vi "test-Implicit-Model-Follower-Test2.vi"(8 "error in (no error)":errorcluster) -> (0 "error out":errorcluster, 3 "All tests passed":bool)   [LabVIEW 2019]
uses:
  <vilib>/Rock Robotics/WPI/ThirdParty/JAS_Junk/TrajLib/LinearSystem_New.vi
  <vilib>/Rock Robotics/WPI/ThirdParty/JAS_Junk/TrajLib/MatBuilder_Create.vi
  <vilib>/Rock Robotics/WPI/ThirdParty/JAS_Junk/TrajLib/MatrixHelper_Zero.vi
  <vilib>/Rock Robotics/WPI/ThirdParty/JAS_Junk/TrajLib/Discretization_DiscretizeAB.vi
  <vilib>/Analysis/baseanly.llb/A x B.vi
  <vilib>/Analysis/baseanly.llb/Real A x B.vi
  <vilib>/Rock Robotics/WPI/ThirdParty/JAS_Junk/TrajLib/MatrixHelper_CoerceSize.vi
  <vilib>/Rock Robotics/WPI/ThirdParty/JAS_Junk/TrajLib/Matrix_Exp.vi
  <vilib>/Rock Robotics/WPI/ThirdParty/JAS_Junk/TrajLib/Matrix_AssignBlock.vi
  <vilib>/Rock Robotics/WPI/ThirdParty/JAS_Junk/TrajLib/Matrix_ExtractFrom.vi
  <vilib>/Analysis/7linalg.llb/Matrix Exp.vi
  <vilib>/Analysis/7linalg.llb/Real Matrix Exp.vi
  <vilib>/Analysis/Matrix/Numeric/Multiply/Multiply.vi
  <vilib>/Analysis/Matrix/Numeric/Multiply/Multiply - RM,R.vi
  <vilib>/Analysis/Matrix/Numeric/Add/Add.vi
  <vilib>/Analysis/Matrix/Numeric/Add/Add - RM,RM.vi
  <vilib>/Rock Robotics/WPI/ThirdParty/JAS_Junk/TrajLib/Trajectory_Library.lvlib
panel:
  out "Test 3":bool
  out "Test 2":bool
  out "Test 1":bool
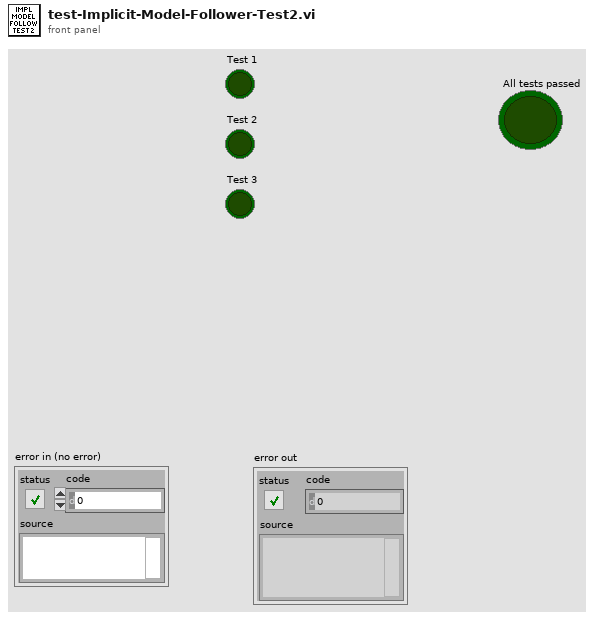
[diagram p1: front panel]
types:
  T1 = typedef "NI_Matrix.lvlib/RealMatrix.ctl" = dbl[][]
  T2 = typedef "Trajectory_Library.lvlib/LINEAR_SYSTEM.ctl" = cluster{"m_A":T1, "m_B":T1, "m_C":T1, "m_D":T1, "States":i32, "Inputs":i32, "Outputs":i32}
  T3 = typedef "Trajectory_Library.lvlib/IMPLICIT_MODEL_FOLLOWER.ctl" = cluster{"m_A":T1, "m_B":T1, "m_U":T1, "States":i32, "Inputs":i32}
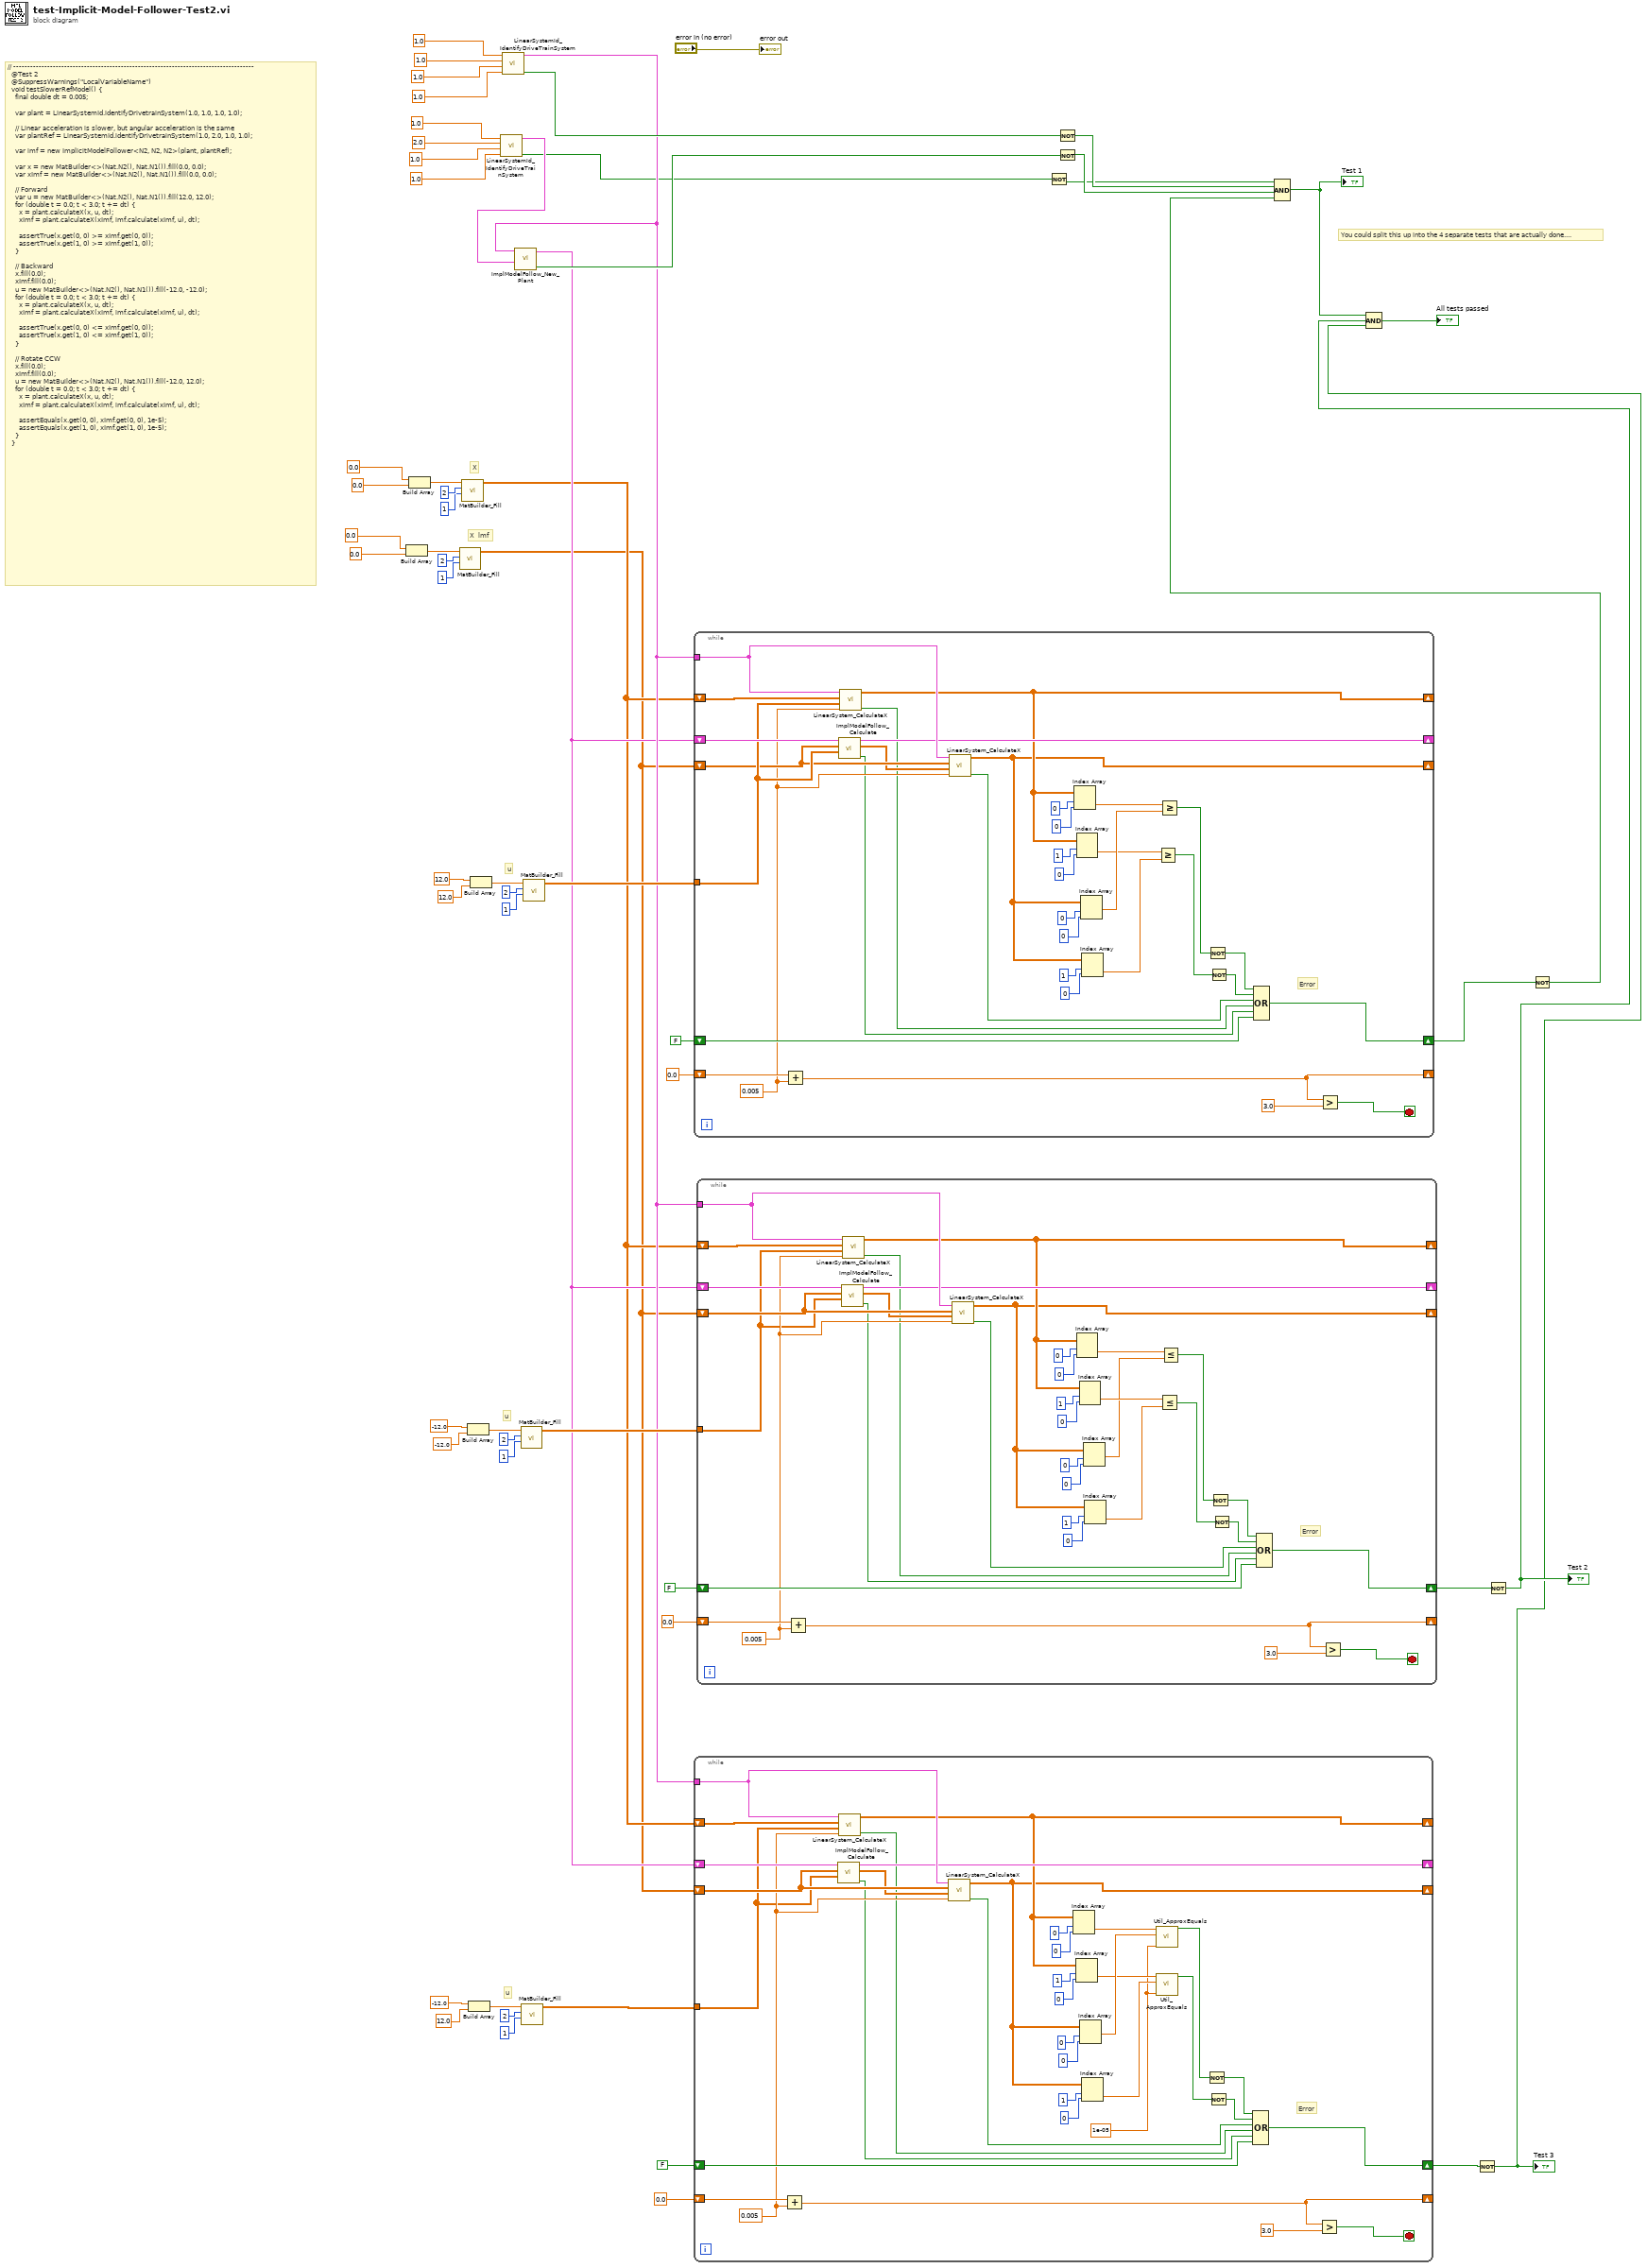
[diagram p0: block diagram]
diagram:
  # "// -------------------------------------------------------------------------------------\n  @Test 2\n  @SuppressWarnings(\"LocalVariableName\")\n  void testSlowerRefModel() {\n    final double dt = 0.005;\n\n    var plant = LinearSystemId.identifyDrivetrainSystem(1.0, 1.0, 1.0, 1.0);\n\n    // Linear acceleration is slower, but angular acceleration is the same\n    var plantRef = LinearSystemId.identifyDrivetrainSystem(1.0, 2.0, 1.0, 1.0);\n\n    var imf = new ImplicitModelFollower<N2, N2, N2>(plant, plantRef);\n\n    var x = new MatBuilder<>(Nat.N2(), Nat.N1()).fill(0.0, 0.0);\n    var xImf = new MatBuilder<>(Nat.N2(), Nat.N1()).fill(0.0, 0.0);\n\n    // Forward\n    var u = new MatBuilder<>(Nat.N2(), Nat.N1()).fill(12.0, 12.0);\n    for (double t = 0.0; t < 3.0; t += dt) {\n      x = plant.calculateX(x, u, dt);\n      xImf = plant.calculateX(xImf, imf.calculate(xImf, u), dt);\n\n      assertTrue(x.get(0, 0) >= xImf.get(0, 0));\n      assertTrue(x.get(1, 0) >= xImf.get(1, 0));\n    }\n\n    // Backward\n    x.fill(0.0);\n    xImf.fill(0.0);\n    u = new MatBuilder<>(Nat.N2(), Nat.N1()).fill(-12.0, -12.0);\n    for (double t = 0.0; t < 3.0; t += dt) {\n      x = plant.calculateX(x, u, dt);\n      xImf = plant.calculateX(xImf, imf.calculate(xImf, u), dt);\n\n      assertTrue(x.get(0, 0) <= xImf.get(0, 0));\n      assertTrue(x.get(1, 0) <= xImf.get(1, 0));\n    }\n\n    // Rotate CCW\n    x.fill(0.0);\n    xImf.fill(0.0);\n    u = new MatBuilder<>(Nat.N2(), Nat.N1()).fill(-12.0, 12.0);\n    for (double t = 0.0; t < 3.0; t += dt) {\n      x = plant.calculateX(x, u, dt);\n      xImf = plant.calculateX(xImf, imf.calculate(xImf, u), dt);\n\n      assertEquals(x.get(0, 0), xImf.get(0, 0), 1e-5);\n      assertEquals(x.get(1, 0), xImf.get(1, 0), 1e-5);\n    }\n  }"
  # "X  lmf"
  # "You could split this up into the 4 separate tests that are actually done...."
  # "u"
  # "u"
  # "u"
  # "X"
  n1 = Build Array(0.0 ("element"), 0.0 ("element")) -> (w31:dbl[])
  n2 = Build Array(0.0 ("element"), 0.0 ("element")) -> (w57:dbl[])
  n3 = call <vilib>:"MatBuilder_Fill.vi"("Columns"=1, "Rows"=2, "Value List"=w31) -> ("output matrix"=w11:T1)  [unwired: 8 in]
  n4 = call <vilib>:"MatBuilder_Fill.vi"("Columns"=1, "Rows"=2, "Value List"=w57) -> ("output matrix"=w12:T1)  [unwired: 8 in]
  n5 = Build Array(-12.0 ("element"), -12.0 ("element")) -> (w41:dbl[])
  n6 = Build Array(-12.0 ("element"), 12.0 ("element")) -> (w36:dbl[])
  n7 = Build Array(12.0 ("element"), 12.0 ("element")) -> (w51:dbl[])
  n8 = call <vilib>:"LinearSystemId_IdentifyDriveTrainSystem.vi"("kAAngular"=1.0 ("rbMeters"), "kVAngular"=1.0 ("rMeters"), "kALinear"=2.0 ("MassKg"), "kVLinear"=1.0 ("JKgMetersSquared")) -> ("Size Coerced"=w1:bool, "Linearsystem"=w3:T2)  [unwired: 6 in]
  n9 = call <vilib>:"LinearSystemId_IdentifyDriveTrainSystem.vi"("kAAngular"=1.0 ("rbMeters"), "kVAngular"=1.0 ("rMeters"), "kALinear"=1.0 ("MassKg"), "kVLinear"=1.0 ("JKgMetersSquared")) -> ("Size Coerced"=w52:bool, "Linearsystem"=w14:T2)  [unwired: 6 in]
  n10 = call <vilib>:"ImplModelFollow_New_Plant.vi"("PlantRef"=w3, "Plant"=w14) -> ("Error"=w26:bool, "IMPLICIT_MODEL_FOLLOWER"=w13:T3)  [unwired: 8 in]
  n11 = call <vilib>:"MatBuilder_Fill.vi"("Columns"=1, "Rows"=2, "Value List"=w41) -> ("output matrix"=w19:T1)  [unwired: 8 in]
  n12 = call <vilib>:"MatBuilder_Fill.vi"("Columns"=1, "Rows"=2, "Value List"=w36) -> ("output matrix"=w15:T1)  [unwired: 8 in]
  n13 = call <vilib>:"MatBuilder_Fill.vi"("Columns"=1, "Rows"=2, "Value List"=w51) -> ("output matrix"=w45:T1)  [unwired: 8 in]
  n14 = while {
    shift-right: [w95] -> _
    shift-left: 0.0 -> [w98]
    tunnel: w14 -> [w85]
    shift-right: [w74] -> _
    shift-left: w12 -> [w94]
    shift-right: [w82] -> w8
    shift-left: FALSE -> [w83]
    shift-right: [w73] -> _
    shift-left: w11 -> [w79]
    shift-right: [w80] -> _
    shift-left: w13 -> [w81]
    tunnel: w15 -> [w64]
    stop <- w97 stop-if-true
    w63 = 1e-05 ("Tolerance")
    w77 = 0.005
    # "Error"
    n15 = Add(x=w98, y=w77) -> (x+y=w95:dbl)
    n16 = call <vilib>:"ImplModelFollow_Calculate.vi"("U"=w64, "X"=w79, "in IMPLICIT_MODEL_FOLLOWER"=w81) -> ("Error"=w75:bool, "U Out"=w78:T1, "out IMPLICIT_MODEL_FOLLOWER"=w80:T3)  [unwired: 6 in]
    n17 = call <vilib>:"LinearSystem_CalculateX.vi"("dT_Seconds"=w77, "ClampedU"=w64, "X"=w94, "Linearsystem"=w85) -> ("Error"=w76:bool, "outX"=w74:T1)  [unwired: 6 in]
    n18 = call <vilib>:"LinearSystem_CalculateX.vi"("dT_Seconds"=w77, "ClampedU"=w78, "X"=w79, "Linearsystem"=w85) -> ("Error"=w84:bool, "outX"=w73:T1)  [unwired: 6 in]
    n19 = Index Array(array=w74, index (row)=0, index (col)=0) -> (element=w72:dbl)
    n20 = Index Array(array=w74, index (row)=1, index (col)=0) -> (element=w70:dbl)
    n21 = Index Array(array=w73, index (row)=0, index (col)=0) -> (element=w71:dbl)
    n22 = Index Array(array=w73, index (row)=1, index (col)=0) -> (element=w69:dbl)
    n23 = call <vilib>:"Util_ApproxEquals.vi"("Tolerance"=w63, "Value 2"=w71, "Value 1"=w72) -> ("ApproxEquals"=w66:bool)  [unwired: 8 in]
    n24 = call <vilib>:"Util_ApproxEquals.vi"("Tolerance"=w63, "Value 2"=w69, "Value 1"=w70) -> ("ApproxEquals"=w65:bool)  [unwired: 8 in]
    n25 = Not(x=w66) -> (.not. x?=w67:bool)
    n26 = Not(x=w65) -> (.not. x?=w68:bool)
    n27 = Compound Arithmetic op=OR(w67, w68, w84, w76, w75, w83) -> (w82:bool)
    n28 = Greater?(x=w95, y=3.0) -> (0:w97:bool)
  }
  n29 = while {
    shift-right: [w130] -> _
    shift-left: 0.0 -> [w133]
    tunnel: w14 -> [w120]
    tunnel: w45 -> [w115]
    shift-right: [w108] -> _
    shift-left: w12 -> [w129]
    shift-right: [w117] -> w43
    shift-left: FALSE -> [w118]
    shift-right: [w107] -> _
    shift-left: w11 -> [w113]
    shift-right: [w114] -> _
    shift-left: w13 -> [w116]
    stop <- w132 stop-if-true
    w111 = 0.005
    # "Error"
    n30 = Add(x=w133, y=w111) -> (x+y=w130:dbl)
    n31 = call <vilib>:"ImplModelFollow_Calculate.vi"("U"=w115, "X"=w113, "in IMPLICIT_MODEL_FOLLOWER"=w116) -> ("Error"=w109:bool, "U Out"=w112:T1, "out IMPLICIT_MODEL_FOLLOWER"=w114:T3)  [unwired: 6 in]
    n32 = call <vilib>:"LinearSystem_CalculateX.vi"("dT_Seconds"=w111, "ClampedU"=w115, "X"=w129, "Linearsystem"=w120) -> ("Error"=w110:bool, "outX"=w108:T1)  [unwired: 6 in]
    n33 = call <vilib>:"LinearSystem_CalculateX.vi"("dT_Seconds"=w111, "ClampedU"=w112, "X"=w113, "Linearsystem"=w120) -> ("Error"=w119:bool, "outX"=w107:T1)  [unwired: 6 in]
    n34 = Index Array(array=w108, index (row)=0, index (col)=0) -> (element=w104:dbl)
    n35 = Index Array(array=w108, index (row)=1, index (col)=0) -> (element=w101:dbl)
    n36 = Index Array(array=w107, index (row)=0, index (col)=0) -> (element=w103:dbl)
    n37 = Index Array(array=w107, index (row)=1, index (col)=0) -> (element=w100:dbl)
    n38 = Greater Or Equal?(x=w101, y=w100) -> (x >= y?=w99:bool)
    n39 = Greater Or Equal?(x=w104, y=w103) -> (x >= y?=w102:bool)
    n40 = Not(x=w102) -> (.not. x?=w105:bool)
    n41 = Not(x=w99) -> (.not. x?=w106:bool)
    n42 = Compound Arithmetic op=OR(w105, w106, w119, w110, w109, w118) -> (w117:bool)
    n43 = Greater?(x=w130, y=3.0) -> (0:w132:bool)
  }
  n44 = while {
    shift-right: [w165] -> _
    shift-left: 0.0 -> [w168]
    tunnel: w14 -> [w155]
    shift-right: [w144] -> _
    shift-left: w12 -> [w164]
    shift-right: [w152] -> w16
    shift-left: FALSE -> [w153]
    shift-right: [w143] -> _
    shift-left: w11 -> [w149]
    shift-right: [w150] -> _
    shift-left: w13 -> [w151]
    tunnel: w19 -> [w140]
    stop <- w167 stop-if-true
    w147 = 0.005
    # "Error"
    n45 = Add(x=w168, y=w147) -> (x+y=w165:dbl)
    n46 = call <vilib>:"ImplModelFollow_Calculate.vi"("U"=w140, "X"=w149, "in IMPLICIT_MODEL_FOLLOWER"=w151) -> ("Error"=w145:bool, "U Out"=w148:T1, "out IMPLICIT_MODEL_FOLLOWER"=w150:T3)  [unwired: 6 in]
    n47 = call <vilib>:"LinearSystem_CalculateX.vi"("dT_Seconds"=w147, "ClampedU"=w140, "X"=w164, "Linearsystem"=w155) -> ("Error"=w146:bool, "outX"=w144:T1)  [unwired: 6 in]
    n48 = call <vilib>:"LinearSystem_CalculateX.vi"("dT_Seconds"=w147, "ClampedU"=w148, "X"=w149, "Linearsystem"=w155) -> ("Error"=w154:bool, "outX"=w143:T1)  [unwired: 6 in]
    n49 = Index Array(array=w144, index (row)=0, index (col)=0) -> (element=w135:dbl)
    n50 = Index Array(array=w144, index (row)=1, index (col)=0) -> (element=w139:dbl)
    n51 = Index Array(array=w143, index (row)=0, index (col)=0) -> (element=w136:dbl)
    n52 = Index Array(array=w143, index (row)=1, index (col)=0) -> (element=w138:dbl)
    n53 = Less Or Equal?(x=w139, y=w138) -> (x <= y?=w137:bool)
    n54 = Less Or Equal?(x=w135, y=w136) -> (x <= y?=w134:bool)
    n55 = Not(x=w134) -> (.not. x?=w141:bool)
    n56 = Not(x=w137) -> (.not. x?=w142:bool)
    n57 = Compound Arithmetic op=OR(w141, w142, w154, w146, w145, w153) -> (w152:bool)
    n58 = Greater?(x=w165, y=3.0) -> (0:w167:bool)
  }
  n59 = Not(x=w1) -> (.not. x?=w2:bool)
  n60 = Not(x=w52) -> (.not. x?=w24:bool)
  n61 = Not(x=w26) -> (.not. x?=w25:bool)
  n62 = Not(x=w8) -> (.not. x?=w20:bool)
  "Test 3" <- w20
  n63 = Not(x=w16) -> (.not. x?=w21:bool)
  "Test 2" <- w21
  n64 = Not(x=w43) -> (.not. x?=w42:bool)
  n65 = Compound Arithmetic op=AND(w2, w24, w25, w42) -> (w23:bool)
  "Test 1" <- w23
  n66 = Compound Arithmetic op=AND(w23, w21, w20) -> (→"All tests passed":bool)
  "error out" <- "error in (no error)"
